vi "Kernel.vi"(0 "ref in":refnum<class "MyPropertyClass_LV2009.lvclass">, 1 "object name":string, 2 "option 1":bool, 3 "option 2":bool, 4 "depth":i32, 5 "error in (no error)":errorcluster, 6 "state":T4, 7 "option 3":bool, 8 "attributes in":variant[](array[variant]), 10 "class attributes in":variant[](array[variant])) -> (11 "class attributes out":variant[](array[variant]), 12 "class hierarchy":T1[](array[typedef]), 13 "attributes out":variant[](array[variant]), 14 "ref out":refnum<class "MyPropertyClass_LV2009.lvclass">, 15 "AttributeRefs":u32[](array[numeric]), 16 "static attribute ref":u32, 17 "output 1":bool, 18 "output 2":bool, 19 "error out":errorcluster)   [LabVIEW 2017, in "MyPropertyClass_LV2009.lvclass"]
doc: "Class kernel, creates and destroys the data value references of the class."
uses:
  MyPropertyClass_LV2009.lvclass
  vi.lib/addons/_AddQ/G#Object/utils/G#Object_State.ctl
  C:/Program Files/National Instruments/LabVIEW 2017/vi.lib/addons/_AddQ/G#Object/G#Object.lvclass
  vi.lib/addons/_AddQ/G#Object/utils/G#Object_ClassHierarchy.ctl
  protected/ClassAttributes.ctl
  protected/ObjectAttributes.ctl
  ClassAttributesRef.ctl
  ObjectAttributesRef.ctl
  MyPropertyClass_LV2009.lvclass/MyPropertyClass_LV2009.ctl
  vi.lib/addons/_AddQ/G#Object/G#Object.lvclass
panel:
  in  "object attributes type":T2
  in  "class attributes type":T3
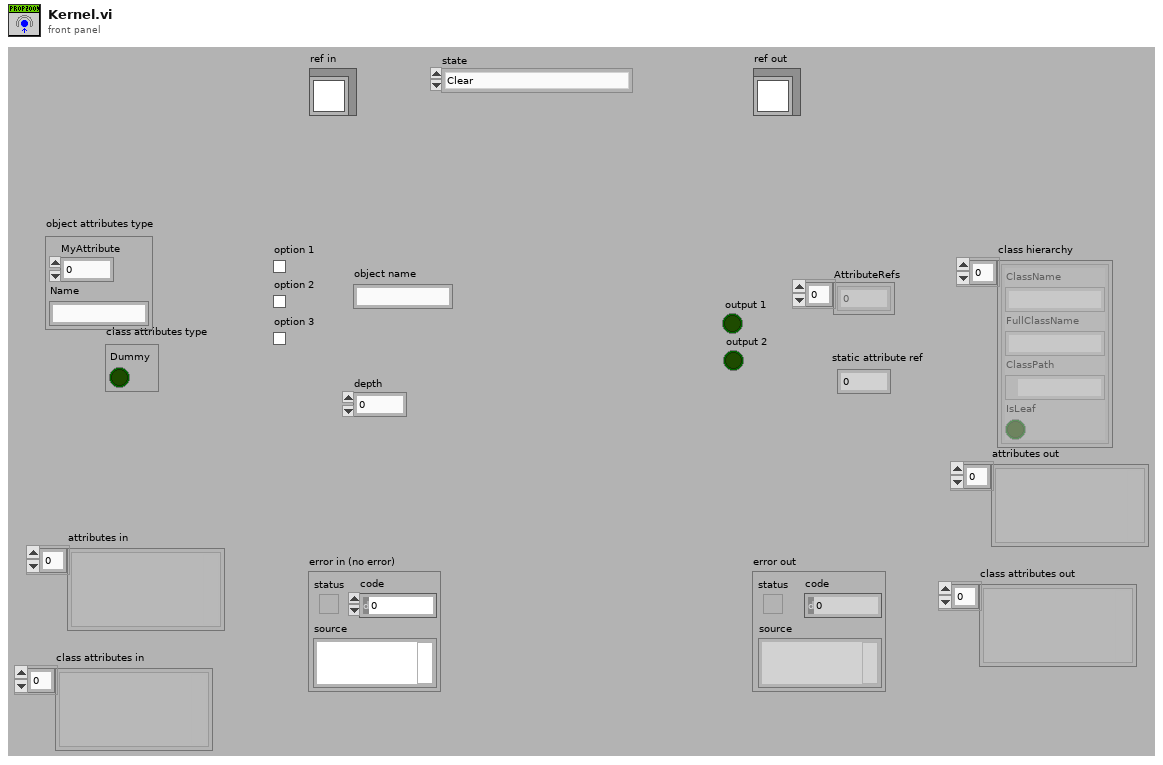
[diagram p1: front panel]
types:
  T1 = typedef "G#Object.lvclass/G#Object_ClassHierarchy.ctl" = cluster{"ClassName":string, "FullClassName":string, "ClassPath":path, "IsLeaf":bool}
  T2 = typedef "MyPropertyClass_LV2009.lvclass/ObjectAttributes.ctl" = cluster{"MyAttribute":dbl, "Name":string}
  T3 = typedef "MyPropertyClass_LV2009.lvclass/ClassAttributes.ctl" = cluster{"Dummy":bool}
  T4 = typedef "G#Object.lvclass/G#Object_State.ctl" = enum16{"Clear", "Create", "Delete", "Get class attributes", "Class hierarchy", "Get attribute value", "Set attribute value"}
  T5 = typedef "MyPropertyClass_LV2009.lvclass/ObjectAttributesRef.ctl" = refnum<data-value>
  T6 = typedef "MyPropertyClass_LV2009.lvclass/ClassAttributesRef.ctl" = refnum<data-value>
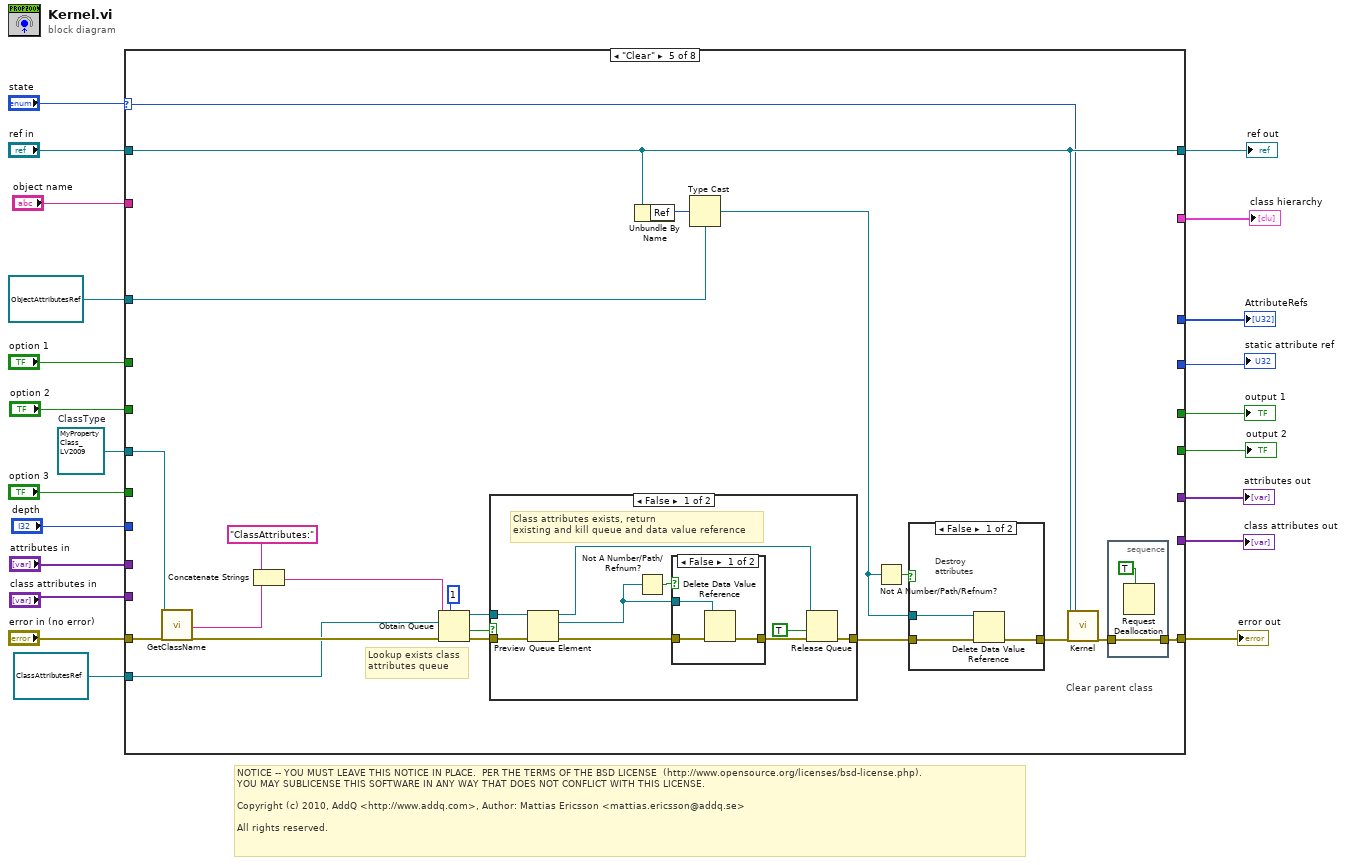
[diagram p0: block diagram]
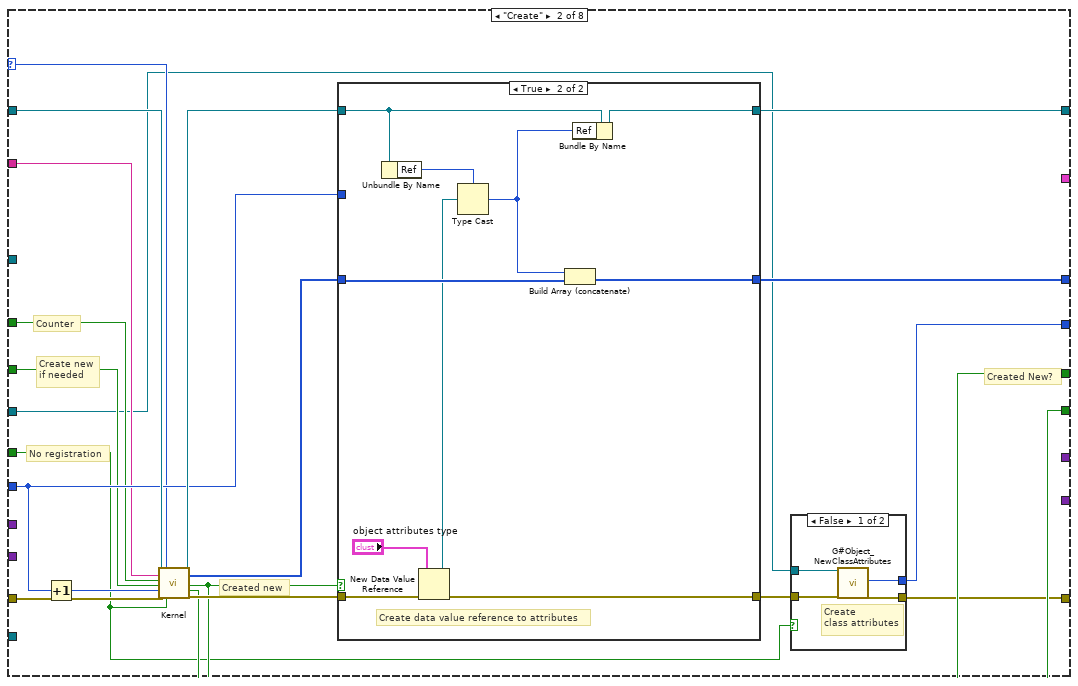
[diagram p3: hidden frame]
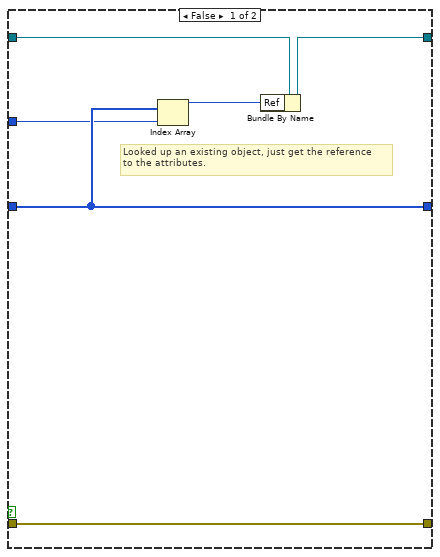
[diagram p5: hidden frame]
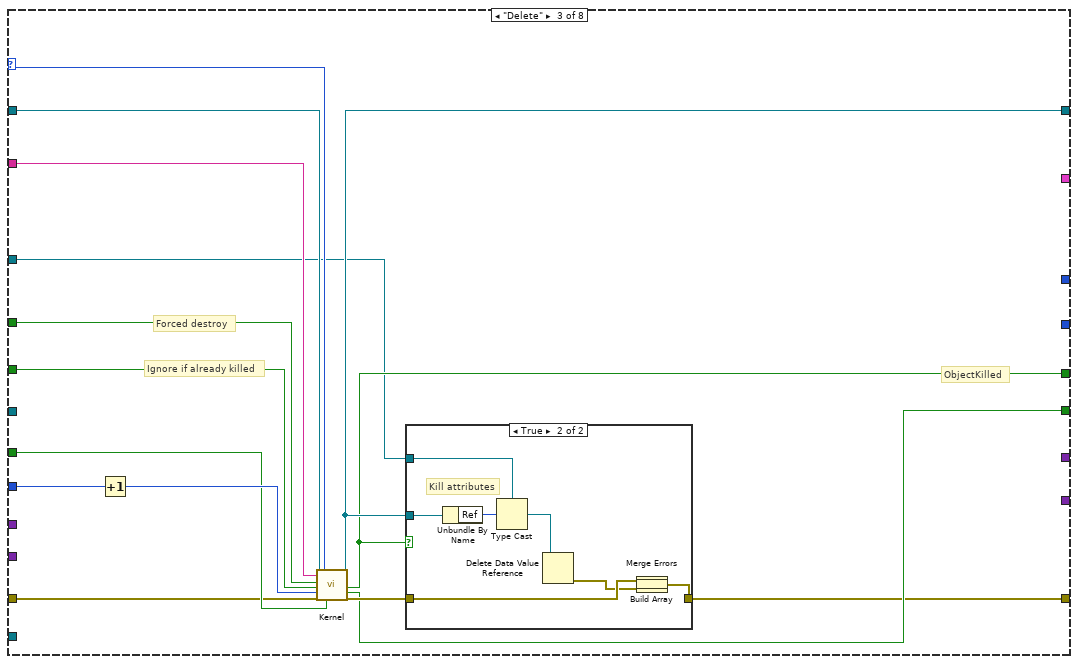
[diagram p6: hidden frame]
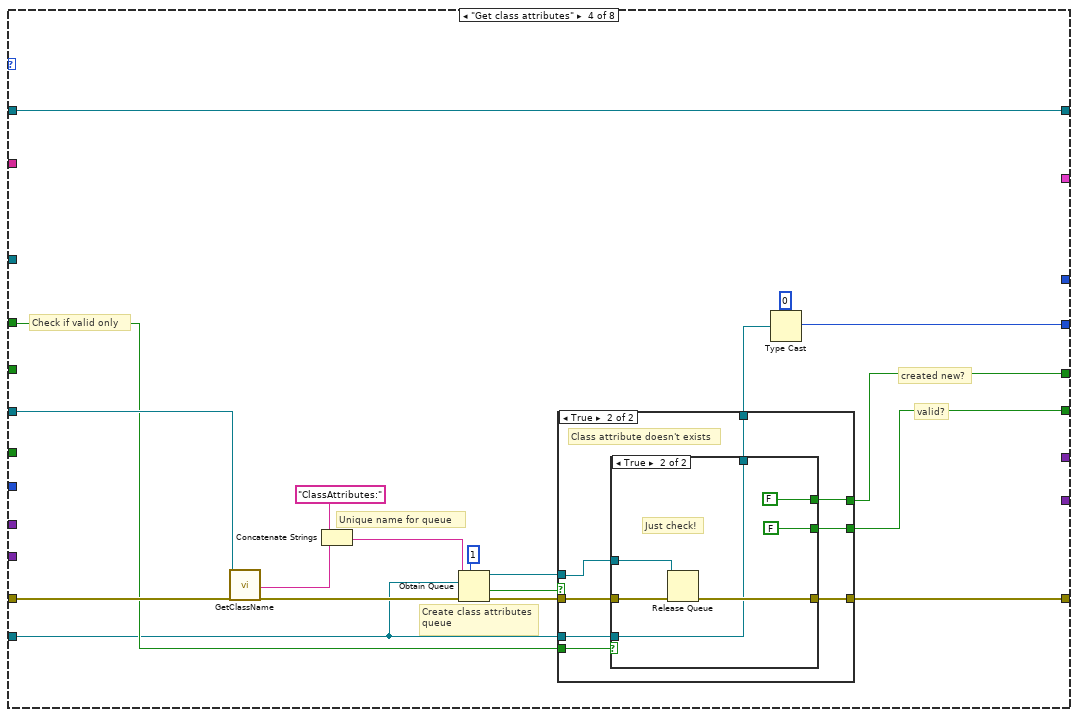
[diagram p8: hidden frame]
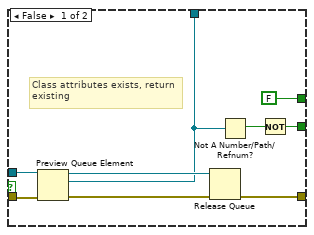
[diagram p9: hidden frame]
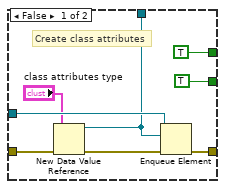
[diagram p10: hidden frame]
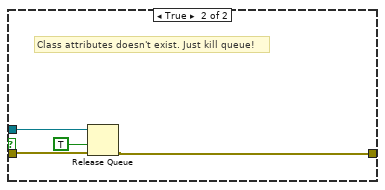
[diagram p13: hidden frame]
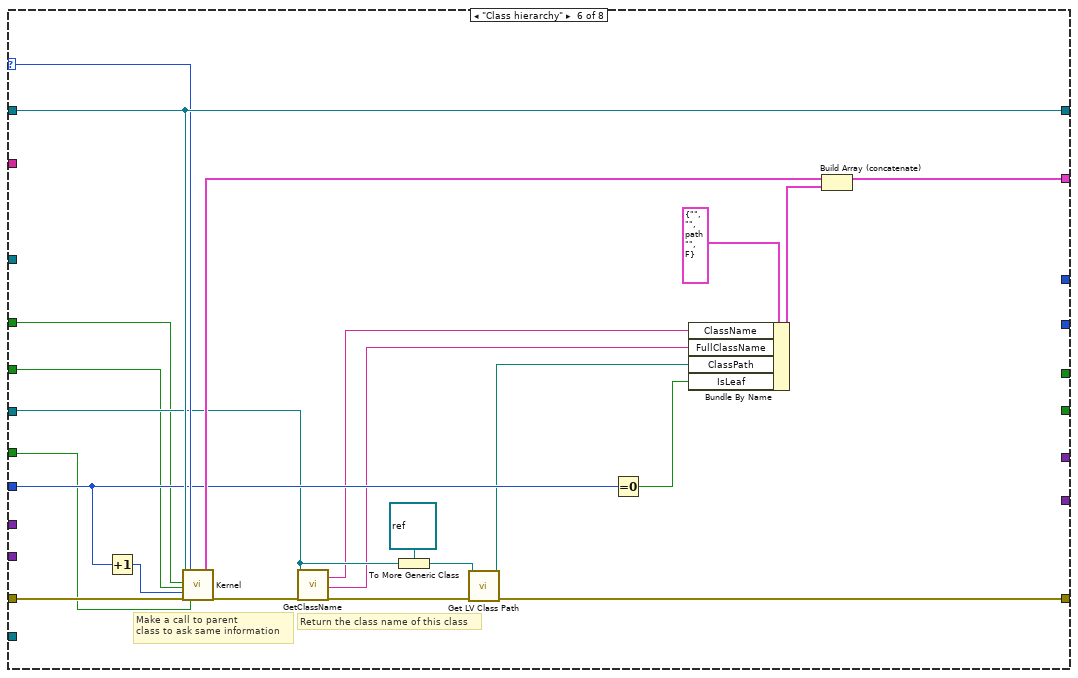
[diagram p14: hidden frame]
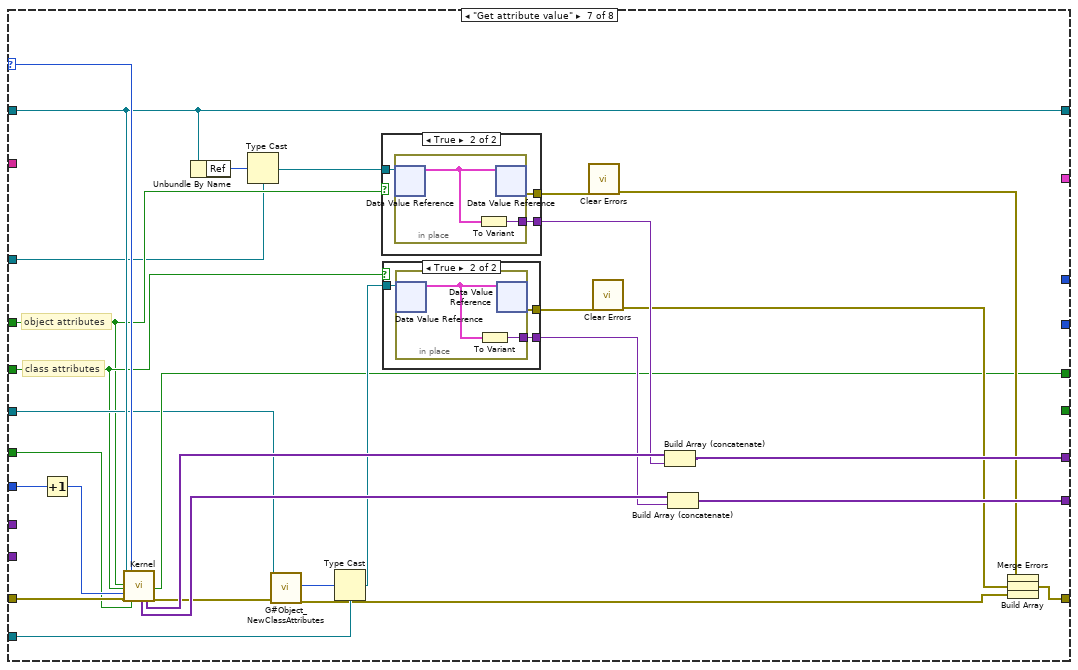
[diagram p15: hidden frame]
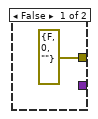
[diagram p16: hidden frame]
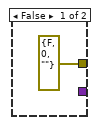
[diagram p17: hidden frame]
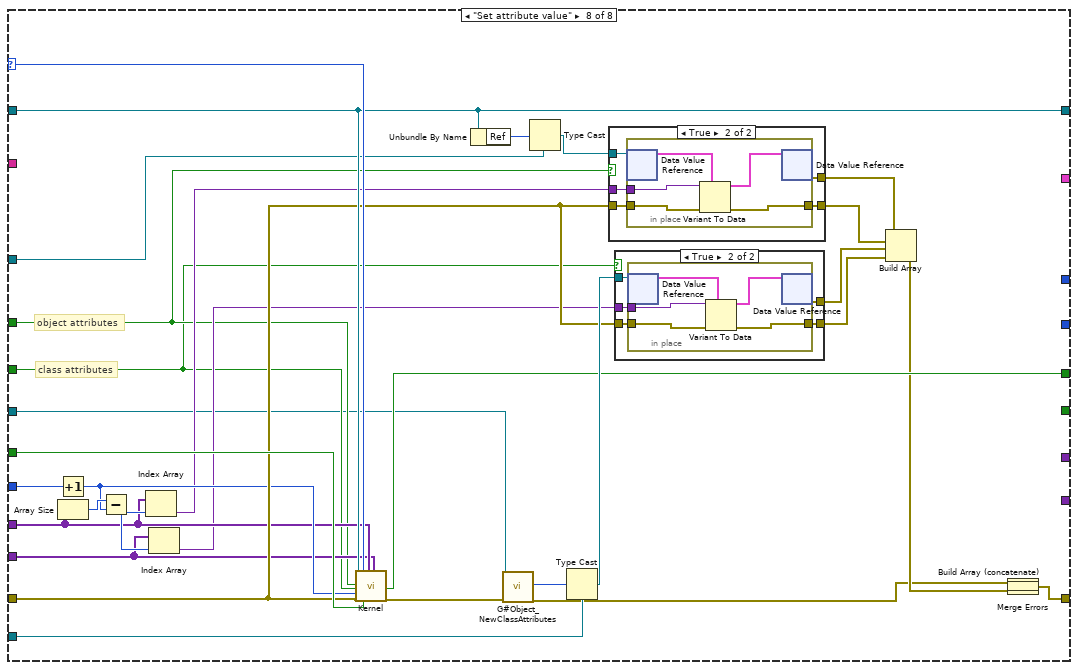
[diagram p18: hidden frame]
diagram:
  w11 = refnum<class "MyPropertyClass_LV2009.lvclass"> refnum  # ClassType
  # "NOTICE -- YOU MUST LEAVE THIS NOTICE IN PLACE.  PER THE TERMS OF THE BSD LICENSE  (http://www.opensource.org/licenses/bsd-license.php).\nYOU MAY SUBLICENSE THIS SOFTWARE IN ANY WAY THAT DOES NOT CONFLICT WITH THIS LICENSE.\n\nCopyright (c) 2010, AddQ <http://www.addq.com>, Author: Mattias Ericsson <mattias.ericsson@addq.se>\n\nAll rights reserved."
  n1 = case shown="\"Clear\"" "state" {
    selector: "state" -> [_ w36 w76 _ w147 w203 w235 w278]
    tunnel: "ref in" -> [w24 w41 w73 w108 w148 w204 w229 w277]
    tunnel: [w24 w40 w79 w108 w148 w204 w229 w277] -> w20
    tunnel: "error in (no error)" -> [w23 w39 w68 w107 w160 w189 w234 w271]
    tunnel: [w23 w26 w67 w97 w143 w187 w226 w276] -> w18
    tunnel: "depth" -> [_ w38 w71 _ _ w196 w219 w265]
    tunnel: "object name" -> [_ w37 w69 _ _ _ _ _]
    tunnel: "option 1" -> [_ w35 w77 w93 _ w186 w210 w257]
    tunnel: [_ w34 _ _ _ _ _ _] -> w14
    tunnel: [_ w32 w78 w90 _ _ w216 w272] -> w13
    tunnel: [_ w27 _ w98 _ _ _ _] -> w12
    tunnel: w11 -> [_ w28 _ w95 w151 w192 w213 w254]
    tunnel: T6 refnum ("data value reference") -> [_ _ _ w92 w150 _ w222 w275]
    tunnel: [_ _ _ _ _ w201 _ _] -> w9
    tunnel: [_ _ _ _ _ _ w231 _] -> w8
    tunnel: [_ _ _ _ _ _ w230 _] -> w7
    tunnel: "option 2" -> [_ w31 w75 _ _ w185 w211 w256]
    tunnel: "option 3" -> [_ w25 w70 _ _ w184 w217 w273]
    tunnel: [_ w30 w74 w91 _ _ _ _] -> w4
    tunnel: "attributes in" -> [_ _ _ _ _ _ _ w261]
    tunnel: "class attributes in" -> [_ _ _ _ _ _ _ w258]
    tunnel: T5 refnum ("attributes ref") -> [_ _ w66 _ w141 _ w208 w249]
    frame Default {
    }
    frame "Create" {
      # "Created new"
      # "No registration"
      # "Create new\nif needed"
      # "Created New?"
      # "Counter"
      n2 = Increment(x=w38) -> (x+1=w33:i32)
      n3 = call-parent "Kernel.vi"("reference in"=w41, "object name"=w37, "option 1"=w35, "option 2"=w31, "depth"=w33, "error in (no error)"=w39, "state"=w36, "option 3"=w25) -> ("reference out"=w42:refnum<class "MyPropertyClass_LV2009.lvclass">, "attribute refs"=w43:u32[], "output 1"=w32:bool, "output 2"=w30:bool, "error out"=w44:errorcluster)  [unwired: 3 in, 4 out]
      n4 = case shown="True" w32 {
        tunnel: w44 -> [w55 w65]
        tunnel: [w55 w59] -> w29
        tunnel: w42 -> [w54 w57]
        tunnel: [w53 w60] -> w40
        tunnel: w43 -> [w52 w63]
        tunnel: [w52 w62] -> w34
        tunnel: w38 -> [w51 _]
        frame False {
          # "Looked up an existing object, just get the reference\nto the attributes."
          # "Already existing"
          n5 = Index Array(array=w52, index=w51) -> (element=w50:u32)
          n6 = Bundle By Name(cluster=w54, "Ref"=w50) -> (w53:refnum<class "MyPropertyClass_LV2009.lvclass">)
        }
        frame True {
          # "Create data value reference to attributes"
          n7 = Unbundle By Name(w57) -> ("Ref"=w56:u32)
          n8 = New Data Value Reference(data value="object attributes type", error in=w65) -> (data value reference=w61:refnum<data-value>, error out=w59:errorcluster)
          n9 = Type Cast(type=w56, x=w61) -> (*(type *) &x=w58:u32)
          n10 = Build Array (concatenate)(w58, w63) -> (w62:u32[])
          n11 = Bundle By Name(cluster=w57, "Ref"=w58) -> (w60:refnum<class "MyPropertyClass_LV2009.lvclass">)
        }
      }
      n12 = case shown="False" w25 {
        tunnel: w29 -> [w48 w49]
        tunnel: w28 -> [w47 _]
        tunnel: [w46 _] -> w27
        tunnel: [w45 w49] -> w26
        frame False {
          # "Create\nclass attributes"
          n13 = call "G#Object_NewClassAttributes.vi"("reference in"=w47, "error in (no error)"=w48) -> ("static attribute ref"=w46:u32, "error out"=w45:errorcluster)  [unwired: 13 in, 3 out]
        }
        frame True {
        }
      }
    }
    frame "Delete" {
      # "Ignore if already killed"
      # "ObjectKilled"
      # "Forced destroy"
      n14 = Increment(x=w71) -> (x+1=w72:i32)
      n15 = call-parent "Kernel.vi"("reference in"=w73, "object name"=w69, "option 1"=w77, "option 2"=w75, "depth"=w72, "error in (no error)"=w68, "state"=w76, "option 3"=w70) -> ("reference out"=w79:refnum<class "MyPropertyClass_LV2009.lvclass">, "output 1"=w78:bool, "output 2"=w74:bool, "error out"=w80:errorcluster)  [unwired: 3 in, 5 out]
      n16 = case shown="True" w78 {
        tunnel: w80 -> [w81 w88]
        tunnel: w79 -> [_ w89]
        tunnel: [w81 w86] -> w67
        tunnel: w66 -> [_ w84]
        frame False {
        }
        frame True {
          # "Kill attributes"
          n17 = Unbundle By Name(w89) -> ("Ref"=w85:u32)
          n18 = Type Cast(type=w84, x=w85) -> (*(type *) &x=w83:T5)
          n19 = Delete Data Value Reference(data value reference=w83) -> (error out=w87:errorcluster)  [unwired: 1 in, 1 out]
          n20 = Build Array(w88, w87) -> (w82:errorcluster[])
          n21 = Merge Errors(w82) -> (w86:errorcluster)
        }
      }
    }
    frame "Get class attributes" {
      # "valid?"
      # "created new?"
      # "Check if valid only"
      # "Unique name for queue"
      # "Create class attributes\nqueue"
      n22 = call-dynamic "GetClassName.vi"("reference in"=w95, "error in (no error)"=w107) -> ("full class name"=w96:string, "error out"=w102:errorcluster)  [unwired: 13 in, 3 out]
      n23 = Concatenate Strings("ClassAttributes:" ("string"), w96) -> (w101:string)
      n24 = Obtain Queue(max queue size (-1, unlimited)=1, name (unnamed)=w101, element data type=w92, error in (no error)=w102) -> (queue out=w103:refnum<queue>, created new?=w94:bool, error out=w104:errorcluster)  [unwired: 1 in]
      n25 = case shown="True" w94 {
        tunnel: w104 -> [w117 w125]
        tunnel: w103 -> [w116 w124]
        tunnel: [w115 w122] -> w97
        tunnel: [w111 w123] -> w99
        tunnel: w93 -> [_ w121]
        tunnel: w92 -> [_ w120]
        tunnel: [w110 w119] -> w91
        tunnel: [FALSE w118] -> w90
        frame False {
          # "Class attributes exists, return\nexisting"
          n26 = Preview Queue Element(queue=w116, error in (no error)=w117) -> (queue out=w113:refnum<queue>, element=w111:T6, error out=w114:errorcluster)  [unwired: 1 in, 1 out]
          n27 = Release Queue(queue=w113, error in (no error)=w114) -> (error out=w115:errorcluster)  [unwired: 1 in, 2 out]
          n28 = Not A Number/Path/Refnum?(number/path/refnum=w111) -> (NaN/Path/Refnum?=w109:bool)
          n29 = Not(x=w109) -> (.not. x?=w110:bool)
        }
        frame True {
          # "Class attribute doesn't exists"
          n30 = case shown="True" w121 {
            tunnel: w125 -> [w133 w139]
            tunnel: w124 -> [w131 w138]
            tunnel: [w130 w136] -> w123
            tunnel: [w129 w137] -> w122
            tunnel: w120 -> [_ w136]
            tunnel: [TRUE FALSE] -> w119
            tunnel: [TRUE FALSE] -> w118
            frame False {
              # "Create class attributes"
              n31 = New Data Value Reference(data value="class attributes type", error in=w133) -> (data value reference=w130:refnum<data-value>, error out=w132:errorcluster)
              n32 = Enqueue Element(queue=w131, element=w130, error in (no error)=w132) -> (error out=w129:errorcluster)  [unwired: 1 in, 2 out]
            }
            frame True {
              # "Just check!"
              n33 = Release Queue(queue=w138, error in (no error)=w139) -> (error out=w137:errorcluster)  [unwired: 1 in, 2 out]
            }
          }
        }
      }
      n34 = Type Cast(type=u32 0, x=w99) -> (*(type *) &x=w98:u32)
    }
    frame "Clear" {
      # "Clear parent class"
      # "Lookup exists class\nattributes queue"
      n35 = call-dynamic "GetClassName.vi"("reference in"=w151, "error in (no error)"=w160) -> ("full class name"=w152:string, "error out"=w154:errorcluster)  [unwired: 13 in, 3 out]
      n36 = Concatenate Strings("ClassAttributes:" ("string"), w152) -> (w153:string)
      n37 = Obtain Queue(max queue size (-1, unlimited)=1, name (unnamed)=w153, element data type=w150, error in (no error)=w154) -> (queue out=w155:refnum<queue>, created new?=w156:bool, error out=w157:errorcluster)  [unwired: 1 in]
      n38 = case shown="False" w156 {
        tunnel: w157 -> [w170 w182]
        tunnel: w155 -> [w171 w183]
        tunnel: [w173 w181] -> w146
        frame False {
          # "Class attributes exists, return\nexisting and kill queue and data value reference"
          n39 = Preview Queue Element(queue=w171, error in (no error)=w170) -> (queue out=w168:refnum<queue>, element=w167:T6, error out=w169:errorcluster)  [unwired: 1 in, 1 out]
          n40 = Not A Number/Path/Refnum?(number/path/refnum=w167) -> (NaN/Path/Refnum?=w174:bool)
          n41 = case shown="False" w174 {
            tunnel: w169 -> [w178 w179]
            tunnel: [w177 w179] -> w172
            tunnel: w167 -> [w176 _]
            frame False {
              n42 = Delete Data Value Reference(data value reference=w176, error in=w178) -> (error out=w177:errorcluster)  [unwired: 1 out]
            }
            frame True {
            }
          }
          n43 = Release Queue(queue=w168, force destroy? (F)=TRUE, error in (no error)=w172) -> (error out=w173:errorcluster)  [unwired: 2 out]
        }
        frame True {
          # "Class attributes doesn't exist. Just kill queue!"
          n44 = Release Queue(queue=w183, force destroy? (F)=TRUE, error in (no error)=w182) -> (error out=w181:errorcluster)  [unwired: 2 out]
        }
      }
      n45 = Unbundle By Name(w148) -> ("Ref"=w142:u32)
      n46 = Type Cast(type=w141, x=w142) -> (*(type *) &x=w140:T5)
      n47 = Not A Number/Path/Refnum?(number/path/refnum=w140) -> (NaN/Path/Refnum?=w149:bool)
      n48 = case shown="False" w149 {
        tunnel: w140 -> [w163 _]
        tunnel: w146 -> [w165 w166]
        tunnel: [w164 w166] -> w145
        frame False {
          # "Destroy\nattributes"
          n49 = Delete Data Value Reference(data value reference=w163, error in=w165) -> (error out=w164:errorcluster)  [unwired: 1 out]
        }
        frame True {
        }
      }
      n50 = call-parent "Kernel.vi"("reference in"=w148, "error in (no error)"=w145, "state"=w147) -> ("error out"=w144:errorcluster)  [unwired: 8 in, 8 out]
      n51 = stacked-sequence {
        tunnel: w144 -> [w161]
        tunnel: [w161] -> w143
        frame #0 {
          n52 = Request Deallocation(TRUE ("flag")) -> ()
        }
      }
    }
    frame "Class hierarchy" {
      # "Make a call to parent\nclass to ask same information"
      # "Return the class name of this class"
      n53 = Increment(x=w196) -> (x+1=w197:i32)
      n54 = call-parent "Kernel.vi"("reference in"=w204, "option 1"=w186, "option 2"=w185, "depth"=w197, "error in (no error)"=w189, "state"=w203, "option 3"=w184) -> ("class hierarchy"=w202:T1[], "error out"=w188:errorcluster)  [unwired: 4 in, 7 out]
      n55 = call-dynamic "GetClassName.vi"("reference in"=w192, "error in (no error)"=w188) -> ("class name"=w190:string, "full class name"=w191:string, "error out"=w193:errorcluster)  [unwired: 13 in, 2 out]
      n56 = To More Generic Class(target class=refnum<class> refnum ("object"), reference=w192) -> (generic class reference=w198:refnum<class>)
      n57 = call <vilib>:"Get LV Class Path.vi"("error in (no error)"=w193, "object"=w198) -> ("error out"=w187:errorcluster, "class path"=w194:path)  [unwired: 8 in]
      n58 = Equal To 0?(x=w196) -> (x = 0?=w195:bool)
      n59 = Bundle By Name(cluster=T1 {"ClassName"="", "FullClassName"="", "ClassPath"=path "", "IsLeaf"=FALSE} ("ClassHierarchy"), "ClassName"=w190, "FullClassName"=w191, "ClassPath"=w194, "IsLeaf"=w195) -> (w199:T1)
      n60 = Build Array (concatenate)(w202, w199) -> (w201:T1[])
    }
    frame "Get attribute value" {
      # "class attributes"
      # "object attributes"
      n61 = Increment(x=w219) -> (x+1=w218:i32)
      n62 = call-parent "Kernel.vi"("reference in"=w229, "option 1"=w210, "option 2"=w211, "depth"=w218, "error in (no error)"=w234, "state"=w235, "option 3"=w217) -> ("class attributes out"=w232:variant[], "attributes out"=w233:variant[], "output 1"=w216:bool, "error out"=w215:errorcluster)  [unwired: 4 in, 5 out]
      n63 = Unbundle By Name(w229) -> ("Ref"=w209:u32)
      n64 = Type Cast(type=w208, x=w209) -> (*(type *) &x=w207:T5)
      n65 = call "G#Object_NewClassAttributes.vi"("reference in"=w213, "error in (no error)"=w215) -> ("static attribute ref"=w212:u32, "error out"=w214:errorcluster)  [unwired: 13 in, 3 out]
      n66 = Type Cast(type=w222, x=w212) -> (*(type *) &x=w221:T6)
      n67 = case shown="True" w210 {
        tunnel: w207 -> [_ w245]
        tunnel: [_ w244] -> w228
        tunnel: [errorcluster {"status"=FALSE, "code"=0, "source"=""} ("error IO") w243] -> w227
        frame False {
        }
        frame True {
          n68 = in-place {
            in-place-border: [w247] -> w244
            n69 = in-place-dvr #1(w245) -> (w246:T2)  [unwired: 1 out]
            n70 = To Variant(anything=w246) -> (Variant=w247:variant)
            n71 = in-place-dvr #1(w246) -> (w243:errorcluster)  [unwired: 1 out]
          }
        }
      }
      n72 = case shown="True" w211 {
        tunnel: [errorcluster {"status"=FALSE, "code"=0, "source"=""} ("error IO") w239] -> w224
        tunnel: w221 -> [_ w238]
        tunnel: [_ w237] -> w220
        frame False {
        }
        frame True {
          n73 = in-place {
            in-place-border: [w241] -> w237
            n74 = in-place-dvr #2(w238) -> (w240:T3)  [unwired: 1 out]
            n75 = To Variant(anything=w240) -> (Variant=w241:variant)
            n76 = in-place-dvr #2(w240) -> (w239:errorcluster)  [unwired: 1 out]
          }
        }
      }
      n77 = call <vilib>:"Clear Errors.vi"("error in (no error)"=w227) -> ("error out"=w225:errorcluster)  [unwired: 5 in, 1 out]
      n78 = call <vilib>:"Clear Errors.vi"("error in (no error)"=w224) -> ("error out"=w223:errorcluster)  [unwired: 5 in, 1 out]
      n79 = Build Array (concatenate)(w233, w228) -> (w231:variant[])
      n80 = Build Array (concatenate)(w232, w220) -> (w230:variant[])
      n81 = Build Array(w225, w223, w214) -> (w206:errorcluster[])
      n82 = Merge Errors(w206) -> (w226:errorcluster)
    }
    frame "Set attribute value" {
      # "class attributes"
      # "object attributes"
      n83 = Increment(x=w265) -> (x+1=w263:i32)
      n84 = Array Size(array=w261) -> (size(s)=w264:i32)
      n85 = Subtract(x=w264, y=w263) -> (x-y=w262:i32)
      n86 = Index Array(array=w261, index=w262) -> (element=w260:variant)
      n87 = Index Array(array=w258, index=w262) -> (element=w259:variant)
      n88 = call-parent "Kernel.vi"("reference in"=w277, "option 1"=w257, "option 2"=w256, "depth"=w263, "error in (no error)"=w271, "state"=w278, "option 3"=w273, "attributes in"=w261, "class attributes in"=w258) -> ("output 1"=w272:bool, "error out"=w255:errorcluster)  [unwired: 2 in, 7 out]
      n89 = Unbundle By Name(w277) -> ("Ref"=w251:u32)
      n90 = call "G#Object_NewClassAttributes.vi"("reference in"=w254, "error in (no error)"=w255) -> ("static attribute ref"=w253:u32, "error out"=w252:errorcluster)  [unwired: 13 in, 3 out]
      n91 = Type Cast(type=w249, x=w251) -> (*(type *) &x=w250:T5)
      n92 = Type Cast(type=w275, x=w253) -> (*(type *) &x=w274:T6)
      n93 = case shown="True" w257 {
        tunnel: w250 -> [_ w284]
        tunnel: w271 -> [w279 w283]
        tunnel: [w279 w282] -> w270
        tunnel: [w279 w281] -> w269
        tunnel: w260 -> [_ w280]
        frame False {
        }
        frame True {
          n94 = in-place {
            in-place-border: w283 -> [w287]
            in-place-border: [w286] -> w281
            in-place-border: w280 -> [w285]
            n95 = in-place-dvr #3(w284) -> (w289:T2)  [unwired: 1 out]
            n96 = Variant To Data(error in=w287, type=w289, Variant=w285) -> (data=w288:T2, error out=w286:errorcluster)
            n97 = in-place-dvr #3(w288) -> (w282:errorcluster)  [unwired: 1 out]
          }
        }
      }
      n98 = case shown="True" w256 {
        tunnel: w274 -> [_ w295]
        tunnel: w271 -> [w290 w294]
        tunnel: [w290 w293] -> w268
        tunnel: [w290 w292] -> w267
        tunnel: w259 -> [_ w291]
        frame False {
        }
        frame True {
          n99 = in-place {
            in-place-border: w294 -> [w298]
            in-place-border: [w297] -> w292
            in-place-border: w291 -> [w296]
            n100 = in-place-dvr #4(w295) -> (w300:T3)  [unwired: 1 out]
            n101 = Variant To Data(error in=w298, type=w300, Variant=w296) -> (data=w299:T3, error out=w297:errorcluster)
            n102 = in-place-dvr #4(w299) -> (w293:errorcluster)  [unwired: 1 out]
          }
        }
      }
      n103 = Build Array(w270, w269, w268, w267) -> (w266:errorcluster[])
      n104 = Build Array (concatenate)(w252, w266) -> (w248:errorcluster[])
      n105 = Merge Errors(w248) -> (w276:errorcluster)
    }
  }
  "error out" <- w18
  "ref out" <- w20
  "AttributeRefs" <- w14
  "static attribute ref" <- w12
  "output 1" <- w13
  "output 2" <- w4
  "class hierarchy" <- w9
  "attributes out" <- w8
  "class attributes out" <- w7
